vi "PreMatch LCD.vi"(5 "Battery Voltage":dbl, 6 "Communication Value:":dbl, 7 "Autonomous Mode":string="ER", 8 "error in":errorcluster, 9 "Camera":dbl, 10 "Distance":dbl, 11 "PSI":dbl) -> (0 "error out":errorcluster)   [LabVIEW 2013]
panel:
  out "Result String 2:":string
  out "Result String 1:":string
  # "0: no camera communication\n1: Camera Communication, not hot goal\n2: Camera Communication, hot goal"
  # "2 Character max!"
  # "0-999"
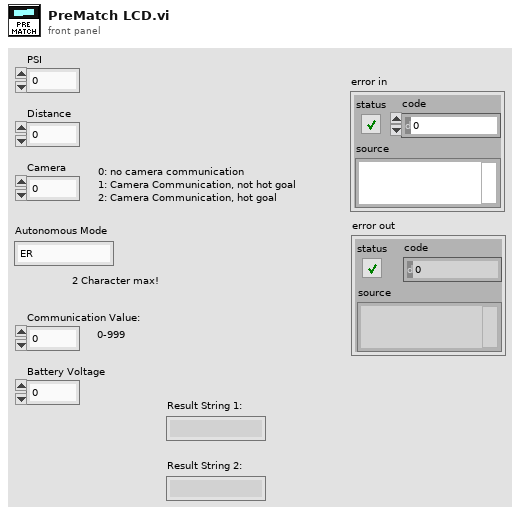
[diagram p1: front panel]
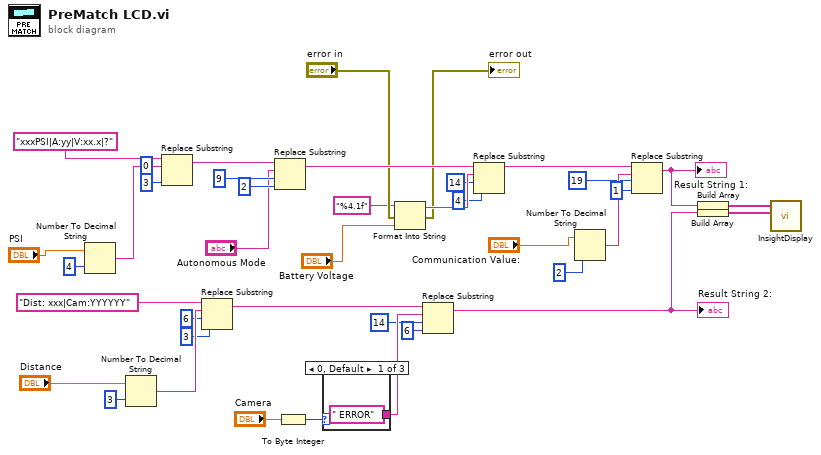
[diagram p0: block diagram]
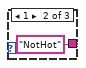
[diagram p2: hidden frame]
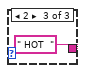
[diagram p3: hidden frame]
diagram:
  n1 = Number To Decimal String(number="PSI", width (-)=i16 4) -> (decimal integer string=w37:string)
  n2 = Number To Decimal String(number="Distance", width (-)=i16 3) -> (decimal integer string=w22:string)
  n3 = Replace Substring(2:3 ("length (len. of substring)"), 3:0 ("offset (0)"), 4:w37, 5:"xxxPSI|A:yy|V:xx.x|?") -> (1:w34:string)  [unwired: 1 out]
  n4 = Replace Substring(2:3 ("length (len. of substring)"), 3:6 ("offset (0)"), 4:w22, 5:"Dist: xxx|Cam:YYYYYY") -> (1:w16:string)  [unwired: 1 out]
  n5 = Replace Substring(2:2 ("length (len. of substring)"), 3:9 ("offset (0)"), 4:"Autonomous Mode", 5:w34) -> (1:w11:string)  [unwired: 1 out]
  n6 = To Byte Integer(number="Camera") -> (8bit integer=w18:i8)
  n7 = case shown="0, Default" w18 {
    tunnel: [" ERROR" "NotHot" " HOT  "] -> w17
    frame 0, Default {
    }
    frame 1 {
    }
    frame 2 {
    }
  }
  n8 = Format Into String(format string="%4.1f", error in="error in", "Battery Voltage") -> (resulting string=w9:string, error out=→"error out":errorcluster)  [unwired: 1 in]
  n9 = Replace Substring(2:6 ("length (len. of substring)"), 3:14 ("offset (0)"), 4:w17, 5:w16) -> (1:w15:string)  [unwired: 1 out]
  "Result String 2:" <- w15
  n10 = Replace Substring(2:4 ("length (len. of substring)"), 3:14 ("offset (0)"), 4:w9, 5:w11) -> (1:w10:string)  [unwired: 1 out]
  n11 = Number To Decimal String(number="Communication Value:", width (-)=i16 2) -> (decimal integer string=w31:string)
  n12 = Replace Substring(2:1 ("length (len. of substring)"), 3:19 ("offset (0)"), 4:w31, 5:w10) -> (1:w26:string)  [unwired: 1 out]
  "Result String 1:" <- w26
  n13 = Build Array(w26) -> (w2:string[])
  n14 = Build Array(w15) -> (w1:string[])
  n15 = call "InsightDisplay.vi"("Zone 2 Data"=w1, "Zone 1 Data"=w2) -> ()  [unwired: 10 in]
